vi "Stop Core.vi"(10 "final error code":i32 caption="code d'erreur final", 11 "Cooler UI with Events in":refnum<class "Cooler UI with Events.lvclass"> caption="Acteur en entrée") -> (3 "Cooler UI with Events out":refnum<class "Cooler UI with Events.lvclass"> caption="Acteur en sortie")   [LabVIEW 2015, in "Cooler UI.lvlib" / "Cooler UI with Events.lvclass"]
doc: "(<B>Nom de fichier</B> : Actor Framework.lvlib:Actor.lvclass:Stop Core.vi)\n\nDéfinit ce que l'acteur fait avant de s'arrêter. Utilisez l'entrée <B>code d'erreur final</B> pour déterminer si l'acteur se ferme en réponse à une erreur.\n\nPar défaut, cette méthode ne fait rien. Une classe descendante peut la redéfinir pour configurer un comportement, tel que la fermeture des processus initialisés par l'acteur dans sa redéfinition de la méthode Noyau d'acteur."
uses:
  Cooler UI with Events.lvclass
  Cooler UI with Events.lvclass/Cooler UI with Events.ctl
  <vilib>/ActorFramework/Actor/Actor.lvclass
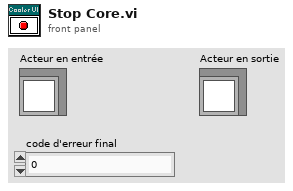
[diagram p1: front panel]
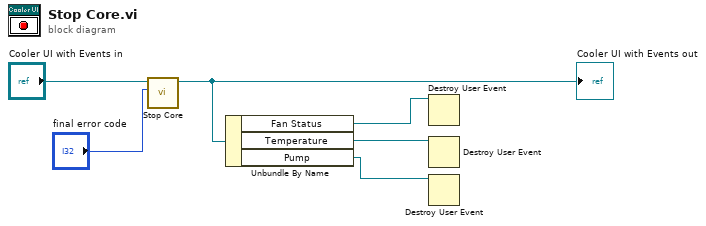
[diagram p0: block diagram]
diagram:
  n1 = call-parent "Stop Core.vi"("final error code"="final error code", "Actor in"="Cooler UI with Events in") -> ("Actor out"=w4:refnum<class "Cooler UI with Events.lvclass">)  [unwired: 9 in]
  "Cooler UI with Events out" <- w4
  n2 = Unbundle By Name(w4) -> ("Fan Status"=w3:refnum<user-event>, "Temperature"=w2:refnum<user-event>, "Pump"=w1:refnum<user-event>)
  n3 = Destroy User Event(user event=w3) -> ()  [unwired: 1 in, 1 out]
  n4 = Destroy User Event(user event=w2) -> ()  [unwired: 1 in, 1 out]
  n5 = Destroy User Event(user event=w1) -> ()  [unwired: 1 in, 1 out]
